vi "DataHandler Type.vi"(8 "error in (no error)":errorcluster, 11 "DataProcessor in":refnum<class "DataProcessor.lvclass">) -> (0 "error out":errorcluster, 2 "DataHandler Type":string, 3 "DataProcessor out":refnum<class "DataProcessor.lvclass">)   [LabVIEW 2020, in "Volatus.lvlib" / "DataProcessor.lvclass"]
uses:
  DataProcessor.lvclass
  DataProcessor.lvclass/DataProcessor.ctl
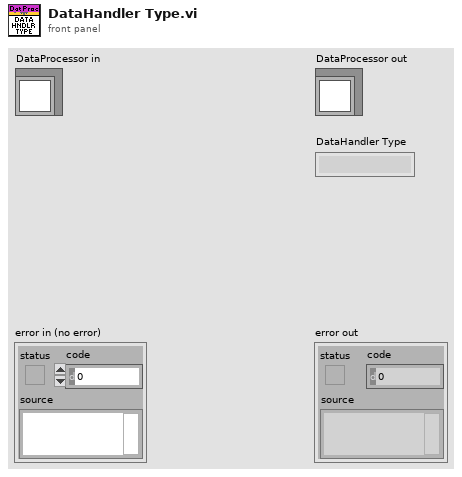
[diagram p1: front panel]
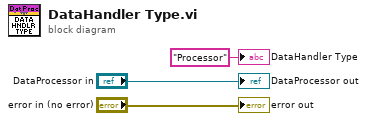
[diagram p0: block diagram]
diagram:
  "error out" <- "error in (no error)"
  "DataProcessor out" <- "DataProcessor in"
  "DataHandler Type" <- "Processor" ("DataHandler Type")
